vi "Intan_ADC_Calibrate.vi"(3 "error in":errorcluster, 5 "VISA resource name":refnum<visa-resource-name>="COM1") -> (0 "error out":errorcluster, 1 "Text response":string, 2 "VISA resource name out":refnum<visa-resource-name>)   [LabVIEW 2020]
doc: "Use this VI to perform ADC self-calibration. This should be called AFTER configuring filters (and other registers)."
panel:
  in  "Teensy event char":string="a"
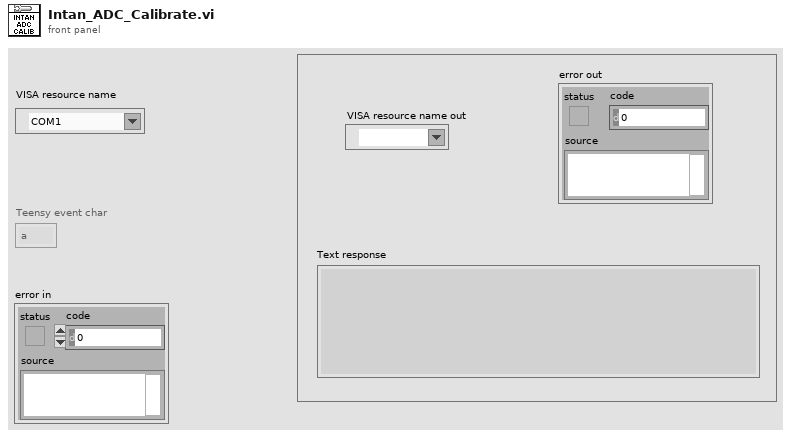
[diagram p1: front panel]
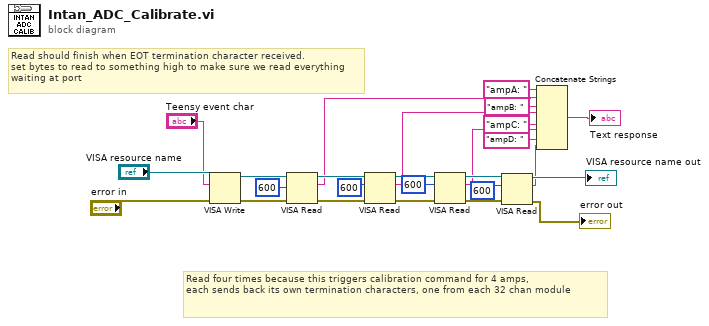
[diagram p0: block diagram]
diagram:
  # "Read four times because this triggers calibration command for 4 amps,\neach sends back its own termination characters, one from each 32 chan module"
  # "Read should finish when EOT termination character received. \nset bytes to read to something high to make sure we read everything waiting at port"
  n1 = VISA Write(VISA resource name="VISA resource name", write buffer="Teensy event char", error in (no error)="error in") -> (VISA resource name out=w23:refnum<visa-resource-name>, error out=w22:errorcluster)  [unwired: 1 out]
  n2 = VISA Read(VISA resource name=w23, byte count=u32 600, error in (no error)=w22) -> (VISA resource name out=w20:refnum<visa-resource-name>, read buffer=w7:string, error out=w19:errorcluster)  [unwired: 1 out]
  n3 = VISA Read(VISA resource name=w20, byte count=u32 600, error in (no error)=w19) -> (VISA resource name out=w16:refnum<visa-resource-name>, read buffer=w4:string, error out=w13:errorcluster)  [unwired: 1 out]
  n4 = VISA Read(VISA resource name=w16, byte count=u32 600, error in (no error)=w13) -> (VISA resource name out=w15:refnum<visa-resource-name>, read buffer=w3:string, error out=w12:errorcluster)  [unwired: 1 out]
  n5 = VISA Read(VISA resource name=w15, byte count=u32 600, error in (no error)=w12) -> (VISA resource name out=→"VISA resource name out":refnum<visa-resource-name>, read buffer=w8:string, error out=→"error out":errorcluster)  [unwired: 1 out]
  n6 = Concatenate Strings("ampA: " ("string"), w7, "ampB: " ("string"), w4, "ampC: " ("string"), w3, "ampD: " ("string"), w8) -> (→"Text response":string)
